vi "6_sub model fitting.vi"(9 "LED I data":dbl[](array[numeric]), 11 "LED V data":dbl[](array[numeric])) -> (1 "LED VI characteristics (regression considering internal resistance)":cluster{dbl[], dbl[]}[](graph), 2 "Regression of LED internal resistance component":cluster{dbl[], dbl[]}[](graph), 3 "LED regression in small current region\nand residual (internal resistance component)":cluster{dbl[], dbl[]}[](graph))   [LabVIEW 2014]
doc: "------------------------------------\nAuther: Koji Ohashi\nCopyright (c) 2020 Japan LabVIEW Users Group, Volunteer members.\nThis VI is released under the MIT License.\nhttp://opensource.org/licenses/mit-license.php\n------------------------------------"
uses:
  <vilib>/Analysis/NI_AALPro.lvlib
panel:
  # "Regression of LED voltage and current data to model formula"
  # "Model formula used for regression analysis"
  # "n: Ideal diode factor\nI0: Reverse saturation current\ne: Napier number\nr: Internal resistance"
  # "e: elementary charge\nk: Boltzmann constant\nT: Absolute temperature"
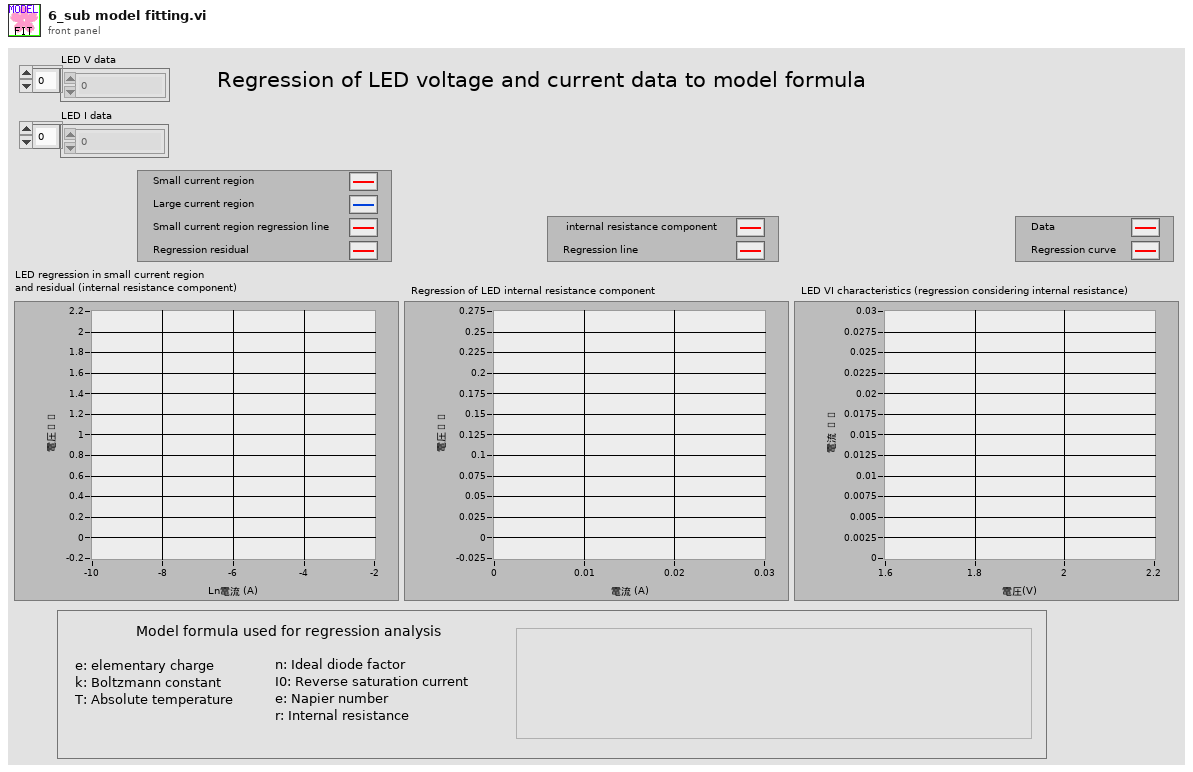
[diagram p1: front panel]
types:
  T1 = cluster{"LED V data":dbl[], "LED I data":dbl[]}[]
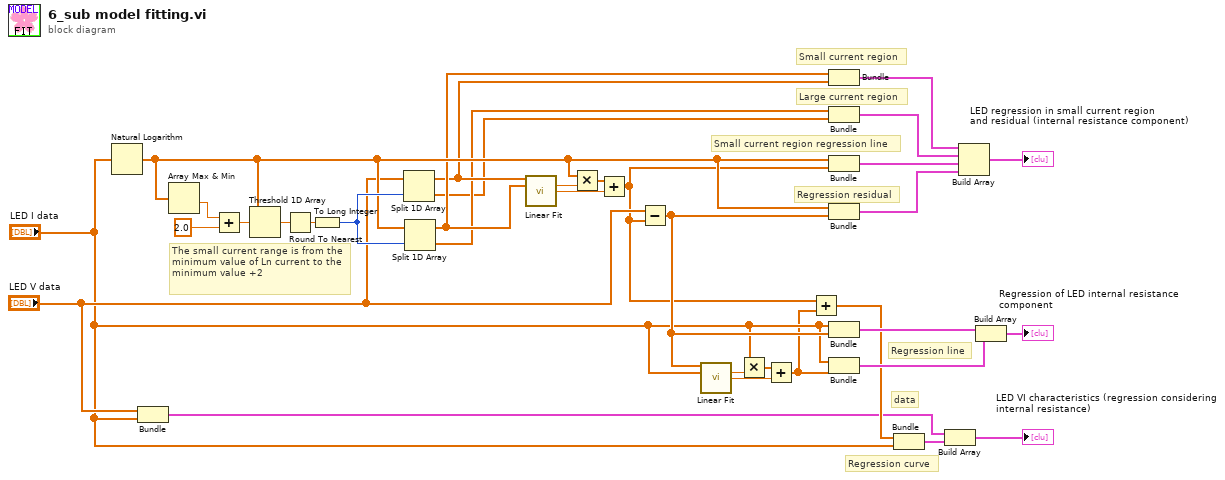
[diagram p0: block diagram]
diagram:
  # "The small current range is from the minimum value of Ln current to the minimum value +2"
  # "Regression curve"
  # "Regression line"
  # "data"
  # "Regression residual"
  # "Small current region regression line"
  # "Large current region"
  # "Small current region"
  n1 = Natural Logarithm(1:"LED I data") -> (0:w12:dbl[])
  n2 = Bundle("LED V data"="LED V data", "LED I data"="LED I data") -> (w5:cluster{"LED V data":dbl[], "LED I data":dbl[]})  [unwired: 1 in]
  n3 = Array Max & Min(array=w12) -> (min value=w21:dbl)  [unwired: 3 out]
  n4 = Add(x=w21, y=2.0) -> (x+y=w19:dbl)
  n5 = Threshold 1D Array(2:w19, 3:w12) -> (0:w18:dbl)  [unwired: 1 in]
  n6 = Round To Nearest(number=w18) -> (nearest integer value=w17:dbl)
  n7 = To Long Integer(number=w17) -> (32bit integer=w13:i32)
  n8 = Split 1D Array(array="LED V data", index=w13) -> (first subarray=w10:dbl[], second subarray=w8:dbl[])
  n9 = Split 1D Array(array=w12, index=w13) -> (first subarray=w11:dbl[], second subarray=w9:dbl[])
  n10 = call <vilib>:"Linear Fit.vi"("Y"=w10, "X"=w11) -> ("slope"=w34:dbl, "intercept"=w32:dbl)  [unwired: 9 in, 3 out]
  n11 = Multiply(x=w12, y=w34) -> (x*y=w33:dbl[])
  n12 = Add(x=w33, y=w32) -> (x+y=w2:dbl[])
  n13 = Subtract(x="LED V data", y=w2) -> (x-y=w26:dbl[])
  n14 = call <vilib>:"Linear Fit.vi"("Y"=w26, "X"="LED I data") -> ("slope"=w24:dbl, "intercept"=w23:dbl)  [unwired: 9 in, 3 out]
  n15 = Multiply(x="LED I data", y=w24) -> (x*y=w25:dbl[])
  n16 = Add(x=w25, y=w23) -> (x+y=w1:dbl[])
  n17 = Add(x=w2, y=w1) -> (x+y=w16:dbl[])
  n18 = Bundle(w11, w10) -> (w7:cluster{dbl[], dbl[]})  [unwired: 1 in]
  n19 = Bundle(w9, w8) -> (w6:cluster{dbl[], dbl[]})  [unwired: 1 in]
  n20 = Bundle(w12, w2) -> (w31:cluster{dbl[], dbl[]})  [unwired: 1 in]
  n21 = Bundle(w12, w26) -> (w29:cluster{dbl[], dbl[]})  [unwired: 1 in]
  n22 = Bundle("LED I data"="LED I data", w26) -> (w27:cluster{"LED I data":dbl[], dbl[]})  [unwired: 1 in]
  n23 = Bundle("LED I data"="LED I data", w1) -> (w22:cluster{"LED I data":dbl[], dbl[]})  [unwired: 1 in]
  n24 = Bundle(w16, "LED I data"="LED I data") -> (w15:cluster{dbl[], "LED I data":dbl[]})  [unwired: 1 in]
  n25 = Build Array(w5, w15) -> (→"LED VI characteristics (regression considering internal resistance)":T1)
  n26 = Build Array(w7, w6, w31, w29) -> (→"LED regression in small current region\nand residual (internal resistance component)":cluster{dbl[], dbl[]}[])
  n27 = Build Array(w27, w22) -> (→"Regression of LED internal resistance component":cluster{"LED I data":dbl[], dbl[]}[])
